vi "Board Remove Player.vi"(8 "error in (no error)":errorcluster, 10 "Player":refnum<class "Player.lvclass">, 11 "Board in":refnum<class "Board.lvclass">) -> (0 "error out":errorcluster, 3 "Board out":refnum<class "Board.lvclass">)   [LabVIEW 2019, in "Board.lvclass"]
uses:
  Board.lvclass
  Player/Player.lvclass
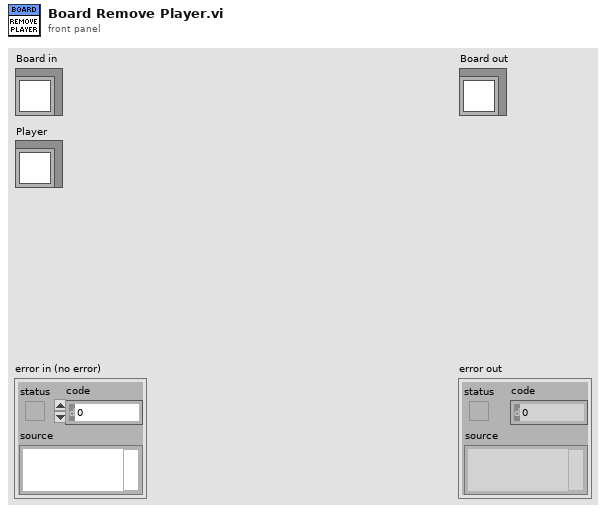
[diagram p1: front panel]
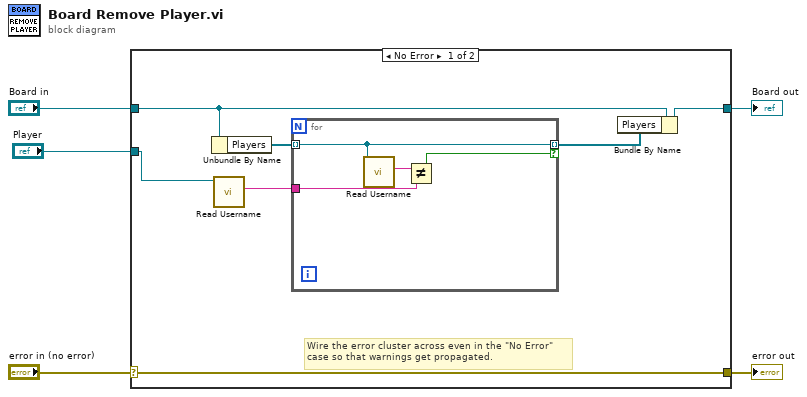
[diagram p0: block diagram]
diagram:
  n1 = case shown="No Error" "error in (no error)" {
    selector: "error in (no error)" -> [w12 w18]
    tunnel: [w12 w18] -> w4
    tunnel: [w7 w17] -> w2
    tunnel: "Board in" -> [w11 w17]
    tunnel: "Player" -> [w9 _]
    frame No Error {
      # "Wire the error cluster across even in the \"No Error\"\ncase so that warnings get propagated."
      n2 = Unbundle By Name(w11) -> ("Players"=w10:refnum<class "Player.lvclass">[])
      n3 = call-dynamic "Read Username.vi"("Player in"=w9) -> ("Username"=w8:string)  [unwired: 8 in, 2 out]
      n4 = for {
        tunnel: w10 -> [w16] mode=indexing
        tunnel: [w16] -> w6 mode=indexing if=w13
        tunnel: w8 -> [w14]
        n5 = call-dynamic "Read Username.vi"("Player in"=w16) -> ("Username"=w15:string)  [unwired: 8 in, 2 out]
        n6 = Not Equal?(x=w15, y=w14) -> (x != y?=w13:bool)
      }
      n7 = Bundle By Name(cluster=w11, "Players"=w6) -> (w7:refnum<class "Board.lvclass">)
    }
    frame Error {
    }
  }
  "error out" <- w4
  "Board out" <- w2
